vi "Unpack Tree Item Open.vi"(11 "TreeItemOpenMsg":refnum<class "TreeItemOpenMsg.lvclass">) -> (0 "Item Tag":string, 1 "Time":u32, 2 "Tree Label":string, 3 "CtlRef":refnum<vi>)   [LabVIEW 2019, in "ActorEvents.lvlib" / "TreeItemOpenMsg.lvclass"]
doc: "<License>\nCopyright © 2017 Composed Systems, LLC | All rights reserved\nwww.composed.io\n\nAuthor: Ethan Stern <ethan.stern@composed.io>\n\nThis software is provided \"AS IS\" WITHOUT WARRANTIES, either express or implied, AND IS FOR EDUCATIONAL PURPOSES ONLY.\n</License>"
uses:
  <vilib>/gpm_packages/@cs/mva-viewable/Source/ActorEvents/IEventAggregator Messages/TreeItemOpenMsg/TreeItemOpenMsg.lvclass
  <vilib>/gpm_packages/@cs/mva-viewable/Source/ActorEvents/IEventAggregator Messages/TreeItemOpenMsg/TreeItemOpenMsg.lvclass/TreeItemOpenMsg.ctl
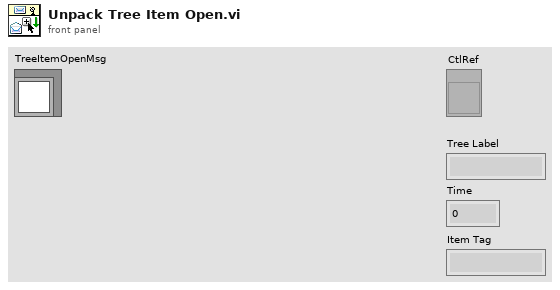
[diagram p1: front panel]
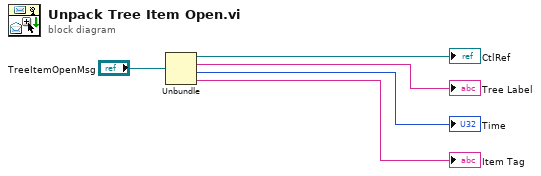
[diagram p0: block diagram]
diagram:
  n1 = Unbundle("TreeItemOpenMsg") -> (→"CtlRef":refnum<vi>, →"Tree Label":string, →"Time":u32, →"Item Tag":string)
